vi "S2C_Shared_Func_Initialize.vi"(8 "Error In":errorcluster, 10 "Func-Q-Name":string, 11 "Cmd-Q-Name":string) -> (0 "Error Out":errorcluster, 2 "Func-Q":refnum<queue>, 3 "Cmd-Q":refnum<queue>)   [LabVIEW 2015]
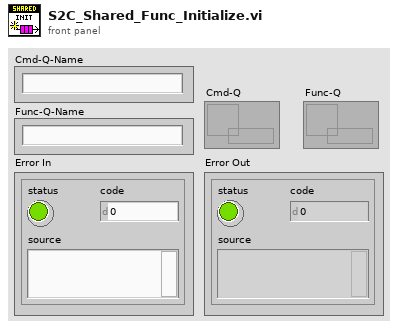
[diagram p1: front panel]
types:
  T1 = cluster{"Caller-Q":refnum<queue>, "Command":string, "Return":string, "Data":variant, "Timeout":dbl}
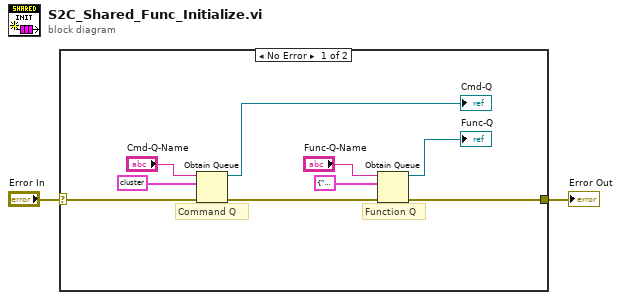
[diagram p0: block diagram]
diagram:
  n1 = case shown="No Error" "Error In" {
    selector: "Error In" -> [w11 w12]
    tunnel: [w5 w12] -> w1
    frame No Error {
      # "Function Q"
      # "Command Q"
      n2 = Obtain Queue(name (unnamed)="Cmd-Q-Name", element data type=T1 {"Caller-Q"=refnum, "Command"="", "Return"="", "Data"=variant, "Timeout"=0.0} ("Command Cluster"), error in (no error)=w11) -> (queue out=→"Cmd-Q":refnum<queue>, error out=w7:errorcluster)  [unwired: 2 in, 1 out]
      n3 = Obtain Queue(name (unnamed)="Func-Q-Name", element data type=cluster{"Command":string, "Response":variant} {"Command"="", "Response"=variant} ("Request Cluster"), error in (no error)=w7) -> (queue out=→"Func-Q":refnum<queue>, error out=w5:errorcluster)  [unwired: 2 in, 1 out]
    }
    frame Error {
    }
  }
  "Error Out" <- w1
